vi "Clear Progress.vi"(8 "error in":errorcluster) -> (0 "error out":errorcluster)   [LabVIEW 2013, in "LVTM.lvlib"]
uses:
  LVTM.lvlib
  Controls_LVTM/Status.ctl
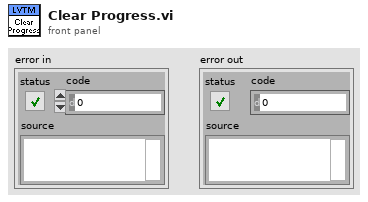
[diagram p1: front panel]
types:
  T1 = typedef "LVTM.lvlib/Status.ctl" = cluster{"Operation":string, "Total Interations":i32, "Current Iteration":i32, "Total Operations":i32, "Current Operation":i32}
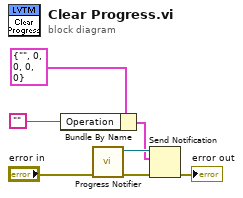
[diagram p0: block diagram]
diagram:
  n1 = Bundle By Name(cluster=T1 {"Operation"="", "Total Interations"=0, "Current Iteration"=0, "Total Operations"=0, "Current Operation"=0} ("notification"), "Operation"="" ("Status (\"\")")) -> (w2:T1)
  n2 = call "Progress Notifier.vi"("error in"="error in") -> ("error out"=w5:errorcluster, "notifier out"=w4:refnum<notifier>)  [unwired: 9 in]
  n3 = Send Notification(notification=w2, notifier=w4, error in (no error)=w5) -> (error out=→"error out":errorcluster)  [unwired: 1 out]
